vi "reset.vi"(8 "error in (no error)":errorcluster, 11 "mbedSerial in":refnum<class "SerialRPC.lvclass">) -> (0 "error out":errorcluster, 3 "mbedSerial out":refnum<class "SerialRPC.lvclass">)   [LabVIEW 2011, in "mbed_LVLibrary.lvlib" / "SerialRPC.lvclass"]
uses:
  SerialRPC.lvclass
  SerialRPC.lvclass/SerialRPC.ctl
  <vilib>/Instr/_visa.llb/VISA Serial Break (Instr).vi
panel:
  # "Reset mbed by sending a break command"
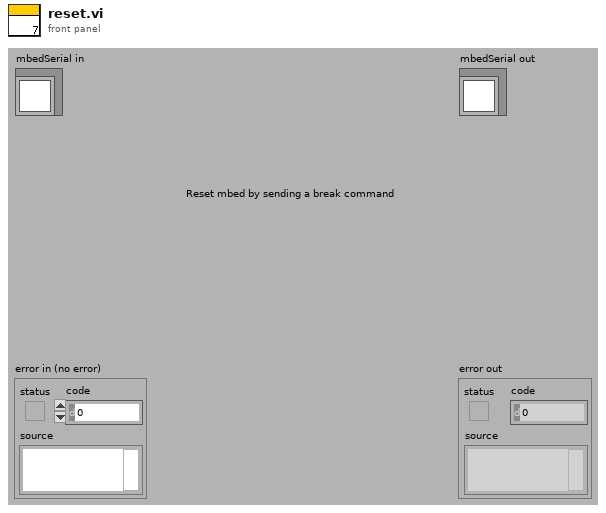
[diagram p1: front panel]
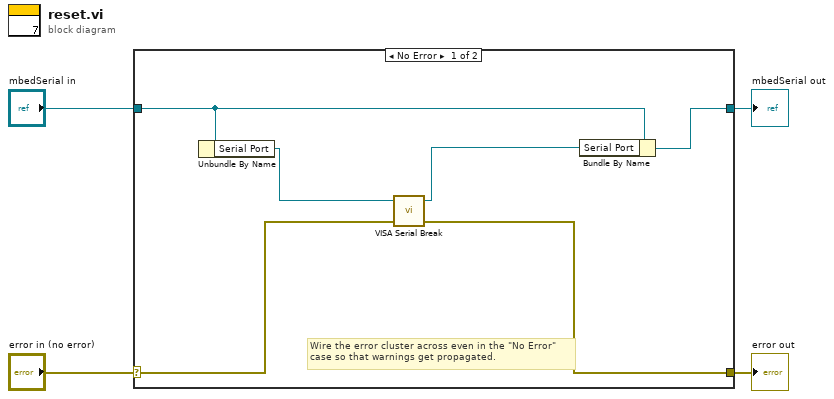
[diagram p0: block diagram]
diagram:
  n1 = case shown="No Error" "error in (no error)" {
    selector: "error in (no error)" -> [w7 w12]
    tunnel: [w6 w12] -> w3
    tunnel: [w9 w11] -> w1
    tunnel: "mbedSerial in" -> [w10 w11]
    frame No Error {
      # "Wire the error cluster across even in the \"No Error\"\ncase so that warnings get propagated."
      n2 = Unbundle By Name(w10) -> ("Serial Port"=w5:refnum<visa-resource-name>)
      n3 = call-poly <vilib>:"VISA Serial Break.vi"("error in (no error)"=w7, "VISA resource name"=w5) -> ("error out"=w6:errorcluster, "VISA resource name out"=w8:refnum<visa-resource-name>)  [unwired: 2 in]
      n4 = Bundle By Name(cluster=w10, "Serial Port"=w8) -> (w9:refnum<class "SerialRPC.lvclass">)
    }
    frame Error {
    }
  }
  "error out" <- w3
  "mbedSerial out" <- w1
